vi "TestExec.Get Seq List.vi"(10 "DefaultSeq":string, 11 "Seq Dir":path) -> (2 "Index":i32, 3 "Seq List":string[](array[string]))   [LabVIEW 2024]
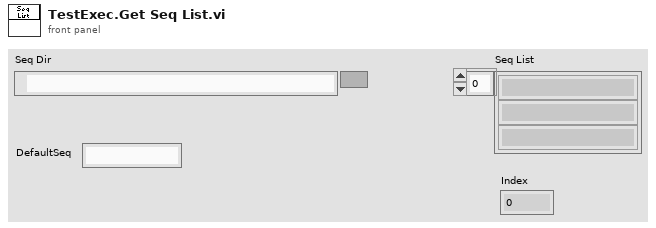
[diagram p1: front panel]
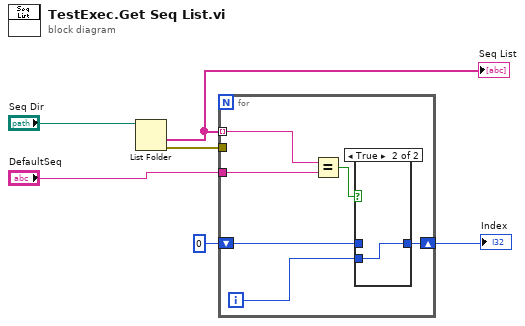
[diagram p0: block diagram]
diagram:
  n1 = List Folder(path="Seq Dir") -> (folder names=w5:string[], error out=w4:errorcluster)  [unwired: 3 in, 2 out]
  "Seq List" <- w5
  n2 = for {
    tunnel: w5 -> [w8] mode=indexing
    shift-right: [w9] -> w2
    shift-left: 0 -> [w11]
    tunnel: w4 -> [_]
    tunnel: "DefaultSeq" -> [w7]
    i -> [w10]
    n3 = Equal?(x=w8, y=w7) -> (x = y?=w12:bool)
    n4 = case shown="True" w12 {
      tunnel: w11 -> [w13 _]
      tunnel: w10 -> [_ w14]
      tunnel: [w13 w14] -> w9
      frame False {
      }
      frame True {
      }
    }
  }
  "Index" <- w2
